vi "Read Element.vi"(8 "error in (no error)":errorcluster, 11 "Array Element 1D in":refnum<class "Vector of Elements.lvclass">) -> (0 "error out":errorcluster, 2 "Element.lvclass":refnum<class "Abs_Type.lvclass">, 3 "Array Element 1D out":refnum<class "Vector of Elements.lvclass">)   [LabVIEW 2019, in "Vector of Elements.lvclass"]
uses:
  Vector of Elements.lvclass
  Type/Abs_Type.lvclass
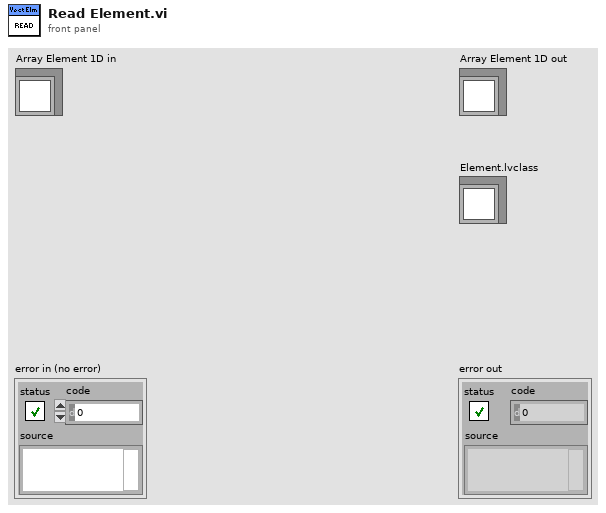
[diagram p1: front panel]
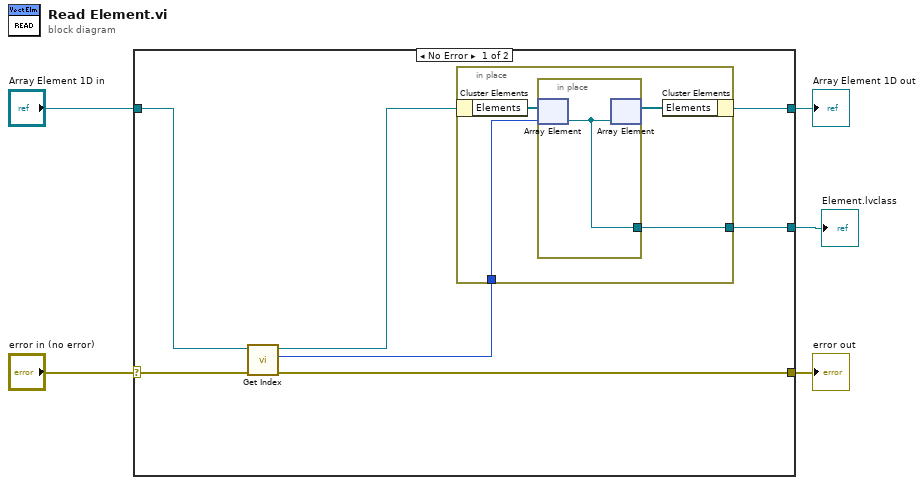
[diagram p0: block diagram]
diagram:
  n1 = case shown="No Error" "error in (no error)" {
    selector: "error in (no error)" -> [w10 w19]
    tunnel: [w8 w19] -> w4
    tunnel: [w11 w18] -> w2
    tunnel: "Array Element 1D in" -> [w9 w18]
    tunnel: [w12 _] -> w1
    frame No Error {
      n2 = call-dynamic "Get Index.vi"("error in (no error)"=w10, "Vector Parent in"=w9) -> ("error out"=w8:errorcluster, "Index"=w6:i32, "Vector Parent out"=w7:refnum<class "Vector of Elements.lvclass">)  [unwired: 7 in]
      n3 = in-place {
        in-place-border: w6 -> [w15]
        in-place-border: [w14] -> w12
        n4 = in-place-cluster #1(w7) -> ("Elements"=w16:refnum<class "Abs_Type.lvclass">[])
        n5 = in-place {
          in-place-border: [w17] -> w14
          n6 = in-place-array #2(w16, w15) -> (w17:refnum<class "Abs_Type.lvclass">)
          n7 = in-place-array #2(w17) -> (w13:refnum<class "Abs_Type.lvclass">[])  [unwired: 1 out]
        }
        n8 = in-place-cluster #1("Elements"=w13) -> (w11:refnum<class "Vector of Elements.lvclass">)
      }
    }
    frame Error {
    }
  }
  "error out" <- w4
  "Array Element 1D out" <- w2
  "Element.lvclass" <- w1
